vi "Intellirupter_coordinated.vi"() -> ()   [LabVIEW 2016]
uses:
  <vilib>/addons/Electrical Power/Protection/Definite Time Delay/subVIs/fpga_Time Delay Cfg.ctl
  <vilib>/FPGAPlugInAG/cRIO-9039 (Sync)/niLvFpga_Open_cRIO-9039 (Sync).vi
  <vilib>/rvi/interface/common/dynamic/niFpgaDynamicAddResources.vi
  <vilib>/Utility/error.llb/Error Cluster From Error Code.vi
  <vilib>/rvi/errors/niLvFpgaAdjustHostInterfaceError.vi
  <vilib>/FPGAPlugInAG/Dynamic/niLvFpga_Close_Dynamic.vi
  <vilib>/rvi/interface/nirviOpenFPGA/nirviOpenFPGA.xnode
  FPGA Bitfiles/IntelliRupter_calibrated.lvbitx
  <vilib>/rvi/interface/nirviReadWriteControl/nirviReadWriteControl.xnode
  <vilib>/rvi/interface/nirviCloseFPGA/nirviCloseFPGA.xnode
  <vilib>/rvi/interface/Simulation/niFpgaSimulationCallBeginRW.vi
  NiFpgaLv.dll
  <vilib>/addons/Electrical Power/Protection/NI_EP_Protection_FPGA.lvlib
panel:
  out "Block Relay8":bool
  out "Block Relay7":bool
  out "Block Relay5":bool
  out "Block Relay4":bool
  out "Block Relay2":bool
  out "Relay8\nBlocking signal":bool[](array[boolean])
  out "Relay7\nBlocking signal":bool[](array[boolean])
  out "Relay5\nBlocking signal":bool[](array[boolean])
  out "Relay4\nBlocking signal":bool[](array[boolean])
  out "Relay2\nBlocking signal":bool[](array[boolean])
  out "Trip Relay8":bool=TRUE
  out "Trip Relay7":bool
  out "Trip Relay6":bool=TRUE
  out "Trip Relay5":bool
  out "Trip Relay4":bool
  out "Trip Relay3":bool=TRUE
  out "Trip Relay2":bool
  out "Trip Relay1":bool
  out "MGCC_to_relay":bool[](array[boolean])=[TRUE, TRUE, FALSE, TRUE, TRUE, FALSE, TRUE, FALSE]
  out "Waveform Chart":dbl(graph)=-0.9071295261383057
  in  "Count(ticks)":u32=10000
  in  "RMS minimum\nvalues":T1={"VRMS values"=[0.5, 0.5, 0.5], "IRMS values"=[0.1, 0.1, 0.1]}
  out "error out":errorcluster
  out "Relay_toMGCC":bool[](array[boolean])=[TRUE, TRUE, FALSE, TRUE, TRUE, FALSE, TRUE, FALSE]
  in  "Manual trip Relay8":bool
  in  "Reclose Relay8?":bool
  out "R8 Data for\ncommunication":dbl[](array[numeric])=[0.0, 2.5009880757512857, 0.03119550342674121, 62.02715630655697, 302.3426407252326, -12.251248359680176, 0.16879604920390107, -0.031540152322164054, 0.0, 0.0]
  in  "Manual trip Relay7":bool
  in  "Reclose Relay7?":bool=TRUE
  out "R7 Data for\ncommunication":dbl[](array[numeric])=[0.0, 2.34510372262792, 2.478950931547994, 62.02269358678421, 62.00633268068818, -0.9071295261383057, 0.09051019032934479, -0.051861350624233596, 0.0, 0.0]
  in  "Manual trip Relay6":bool
  in  "Reclose Relay6?":bool
  out "R6 Data for\ncommunication":dbl[](array[numeric])=[0.0, 2.348051907862318, 0.01545718535019481, 62.01511039984677, 317.9551888289113, -12.64305591583252, 0.014835873481385646, -0.011305832700669725, 0.0, 0.0]
  in  "Manual trip Relay5":bool
  in  "Reclose Relay5?":bool=TRUE
  out "R5 Data for\ncommunication":dbl[](array[numeric])=[1.0, 2.346495418202577, 2.356958918684434, 62.01843298132032, 62.025906318306994, -0.8903157114982605, -0.5565142908906333, -0.4184036072959372, 0.0, 0.0]
  in  "Manual trip Relay4":bool
  in  "Reclose Relay4?":bool=TRUE
  out "R4 Data for\ncommunication":dbl[](array[numeric])=[1.0, 2.35949711967503, 2.3520019383369224, 62.03276424249066, 62.0133797943195, -0.28130459785461426, 0.5952503478367136, 0.39746847420084586, 0.0, 0.0]
  in  "Manual trip Relay3":bool
  in  "Reclose Relay3?":bool
  out "R3 Data for\ncommunication":dbl[](array[numeric])=[0.0, 2.3645958826384064, 0.01384802207001256, 62.02232220042387, 281.0580123337938, 37.610870361328125, 0.01240386848085533, 0.025416571188110054, 0.0, 0.0]
  in  "Manual trip Relay2":bool
  in  "Reclose Relay2?":bool=TRUE
  out "R2 Data for\ncommunication":dbl[](array[numeric])=[1.0, 2.35591902204862, 2.357236343046619, 62.02966341388489, 62.010588677473145, 0.21399852633476257, 1.122459889869548, 0.5804481897422749, 0.0, 0.0]
  out "R1 Data for\ncommunication":dbl[](array[numeric])=[1.0, 2.364986795195867, 2.3598010106583396, 62.02800601231562, 62.01433053877221, 0.17643588781356812, 1.6919416172136679, 0.8721834487461031, 0.0, 0.0]
  in  "Relay8":bool
  in  "Relay7":bool
  in  "Relay6":bool
  in  "Relay5":bool=TRUE
  in  "Relay4":bool=TRUE
  in  "Relay3":bool
  in  "Relay2":bool=TRUE
  in  "Reclose Relay1?":bool=TRUE
  out "half cycle (samples)":i32=96
  out "basic calc interval":u16=2074
  in  "stop":bool
  in  "Relay1":bool=TRUE
  in  "Manual trip Relay1":bool
  # "status\nmag_left\nmag_right\nfreq_left\nfreq_right\nang_diff\nact_power\nrea_power\n0\n0"
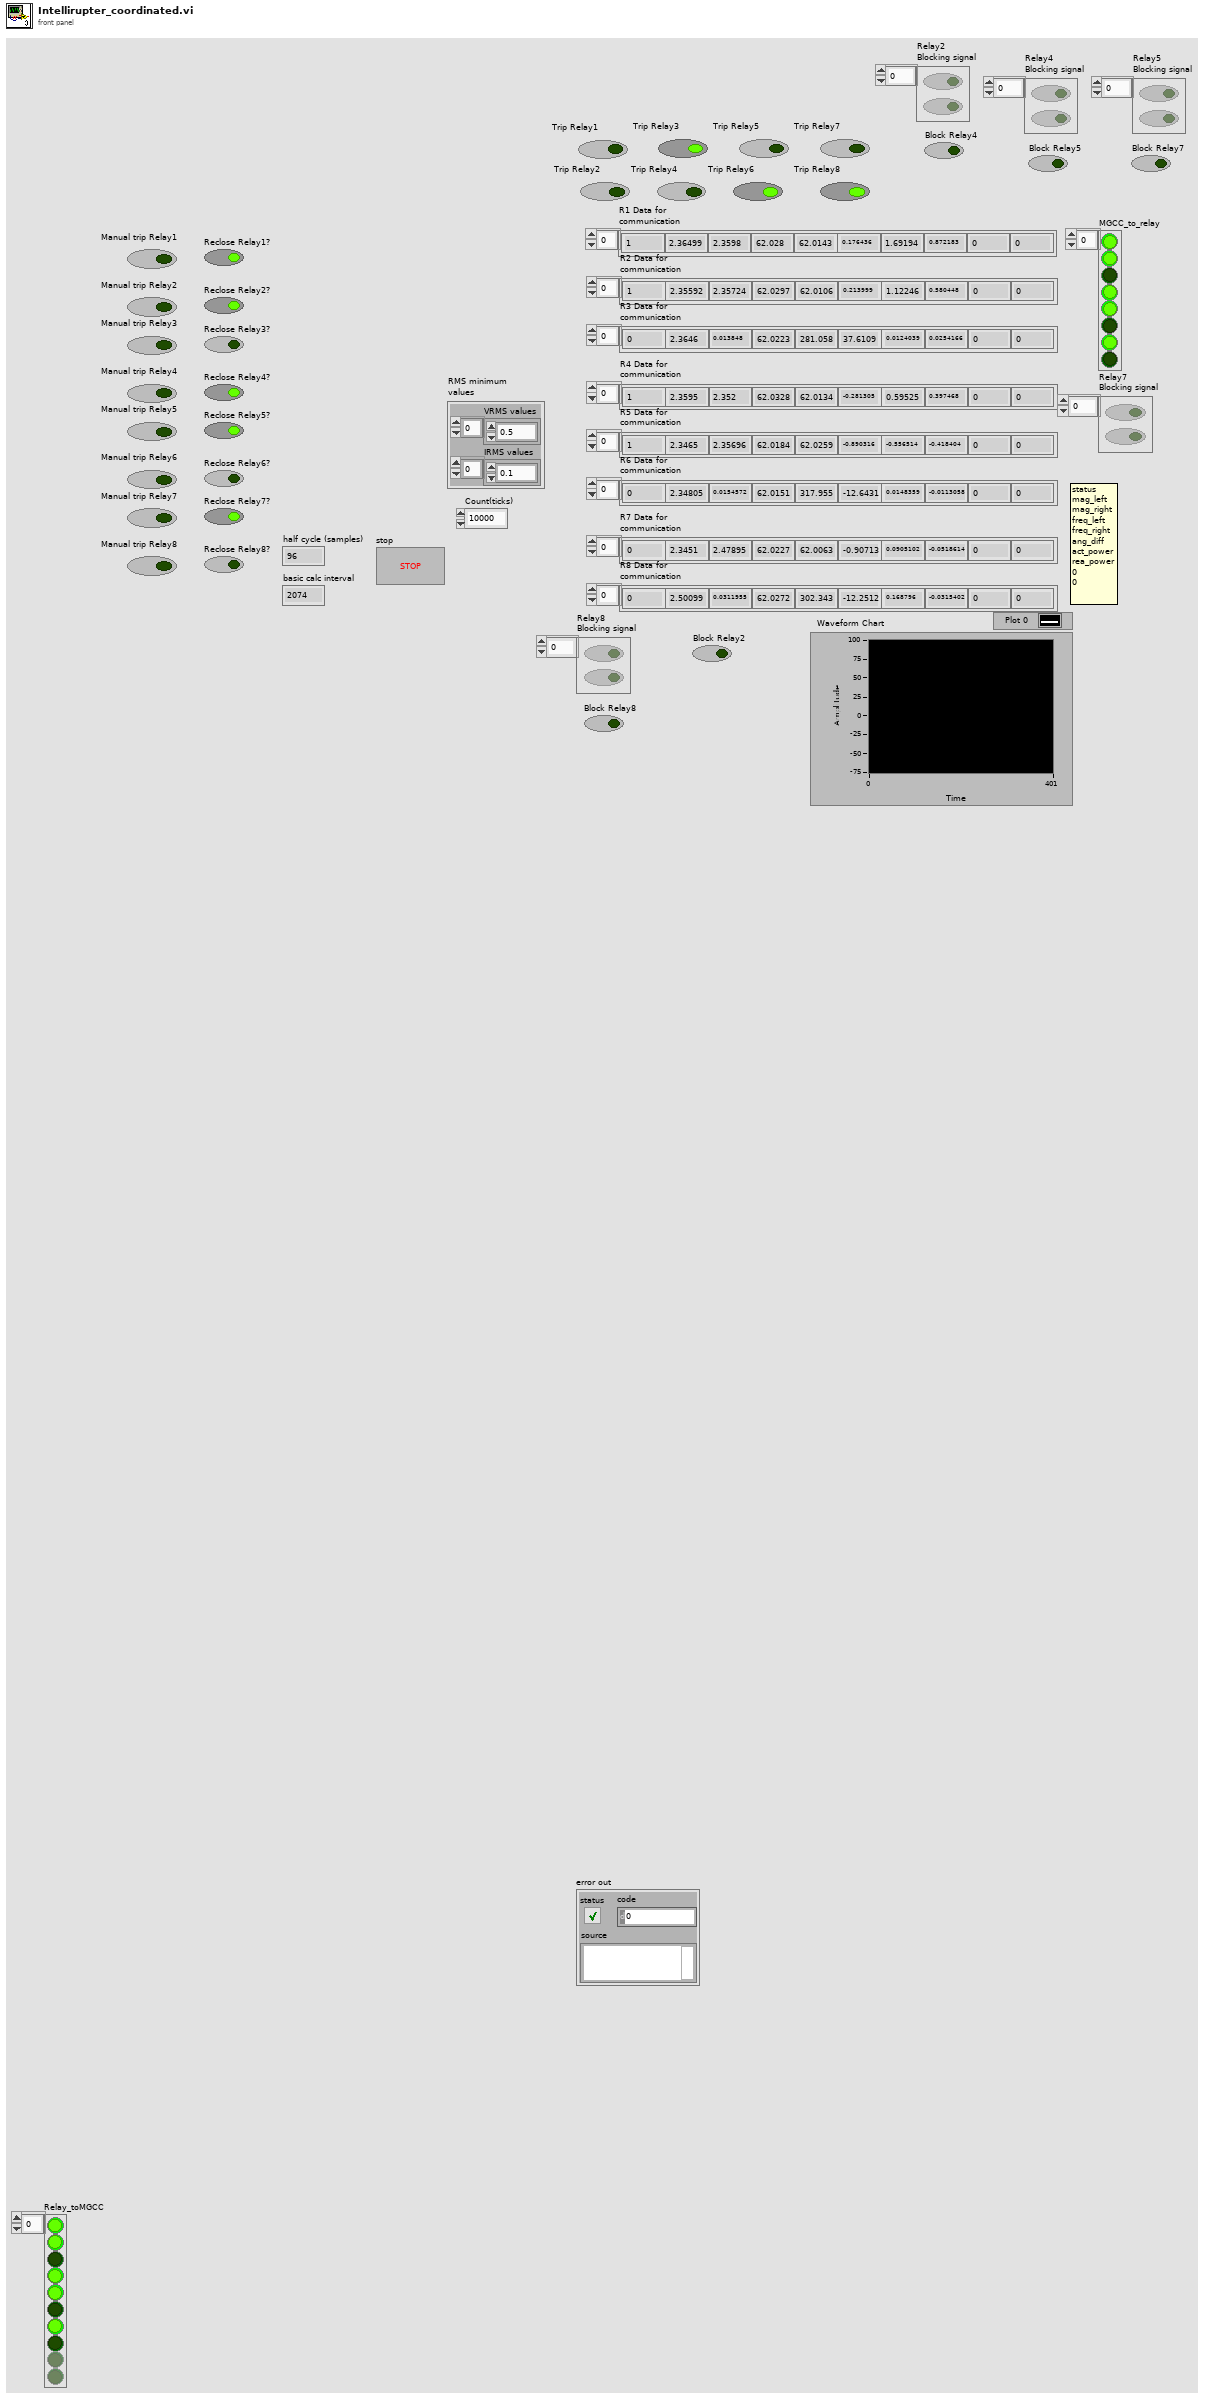
[diagram p1: front panel]
types:
  T1 = cluster{"VRMS values":dbl[], "IRMS values":dbl[]}
  T2 = cluster{fxp<+/-,53,11>[], fxp<+/-,53,11>[], fxp<+/-,53,11>[], fxp<+/-,53,11>[], fxp<+/-,53,11>[], fxp<+/-,53,11>[], fxp<+/-,53,11>[], fxp<+/-,53,11>[], fxp<+/-,53,11>[]}
  T3 = typedef "NI_EP_Protection_FPGA.lvlib/fpga_Time Delay Cfg.ctl" = cluster{"operate time [ms]":u32, "reset time [ms]":u32, "operate time compensation [ms]":u32}
  T4 = cluster{"UV Reset level":dbl, "Undervoltage \npick-up level":dbl, "OC Reset level":dbl, "Overcurrent\npick-up level":dbl, "time delay settings":T3}
  T5 = cluster{"Magnitude Minimum":dbl, "Magnitude difference level":dbl, "Frequency difference level":dbl, "Phase difference level":dbl}
  T6 = cluster{"RMS values":dbl[], "RMS values":dbl[], "RMS values":dbl[]}
  T7 = typedef "NI_EP_Protection_FPGA.lvlib/fpga_Timer Feedback Var.ctl" = cluster{"time elapsed":u32, "start time of trip counting":u32, "start time of reseting":u32}
  T8 = typedef "NI_EP_Protection_FPGA.lvlib/fpga_State.ctl" = enum16{"Idle", "Trip Counting", "Tripped", "Reset Counting"}
  T9 = cluster{bool, bool, "Boolean":bool, "timing values out":T7, "status out":T8, "trip signal out":bool}
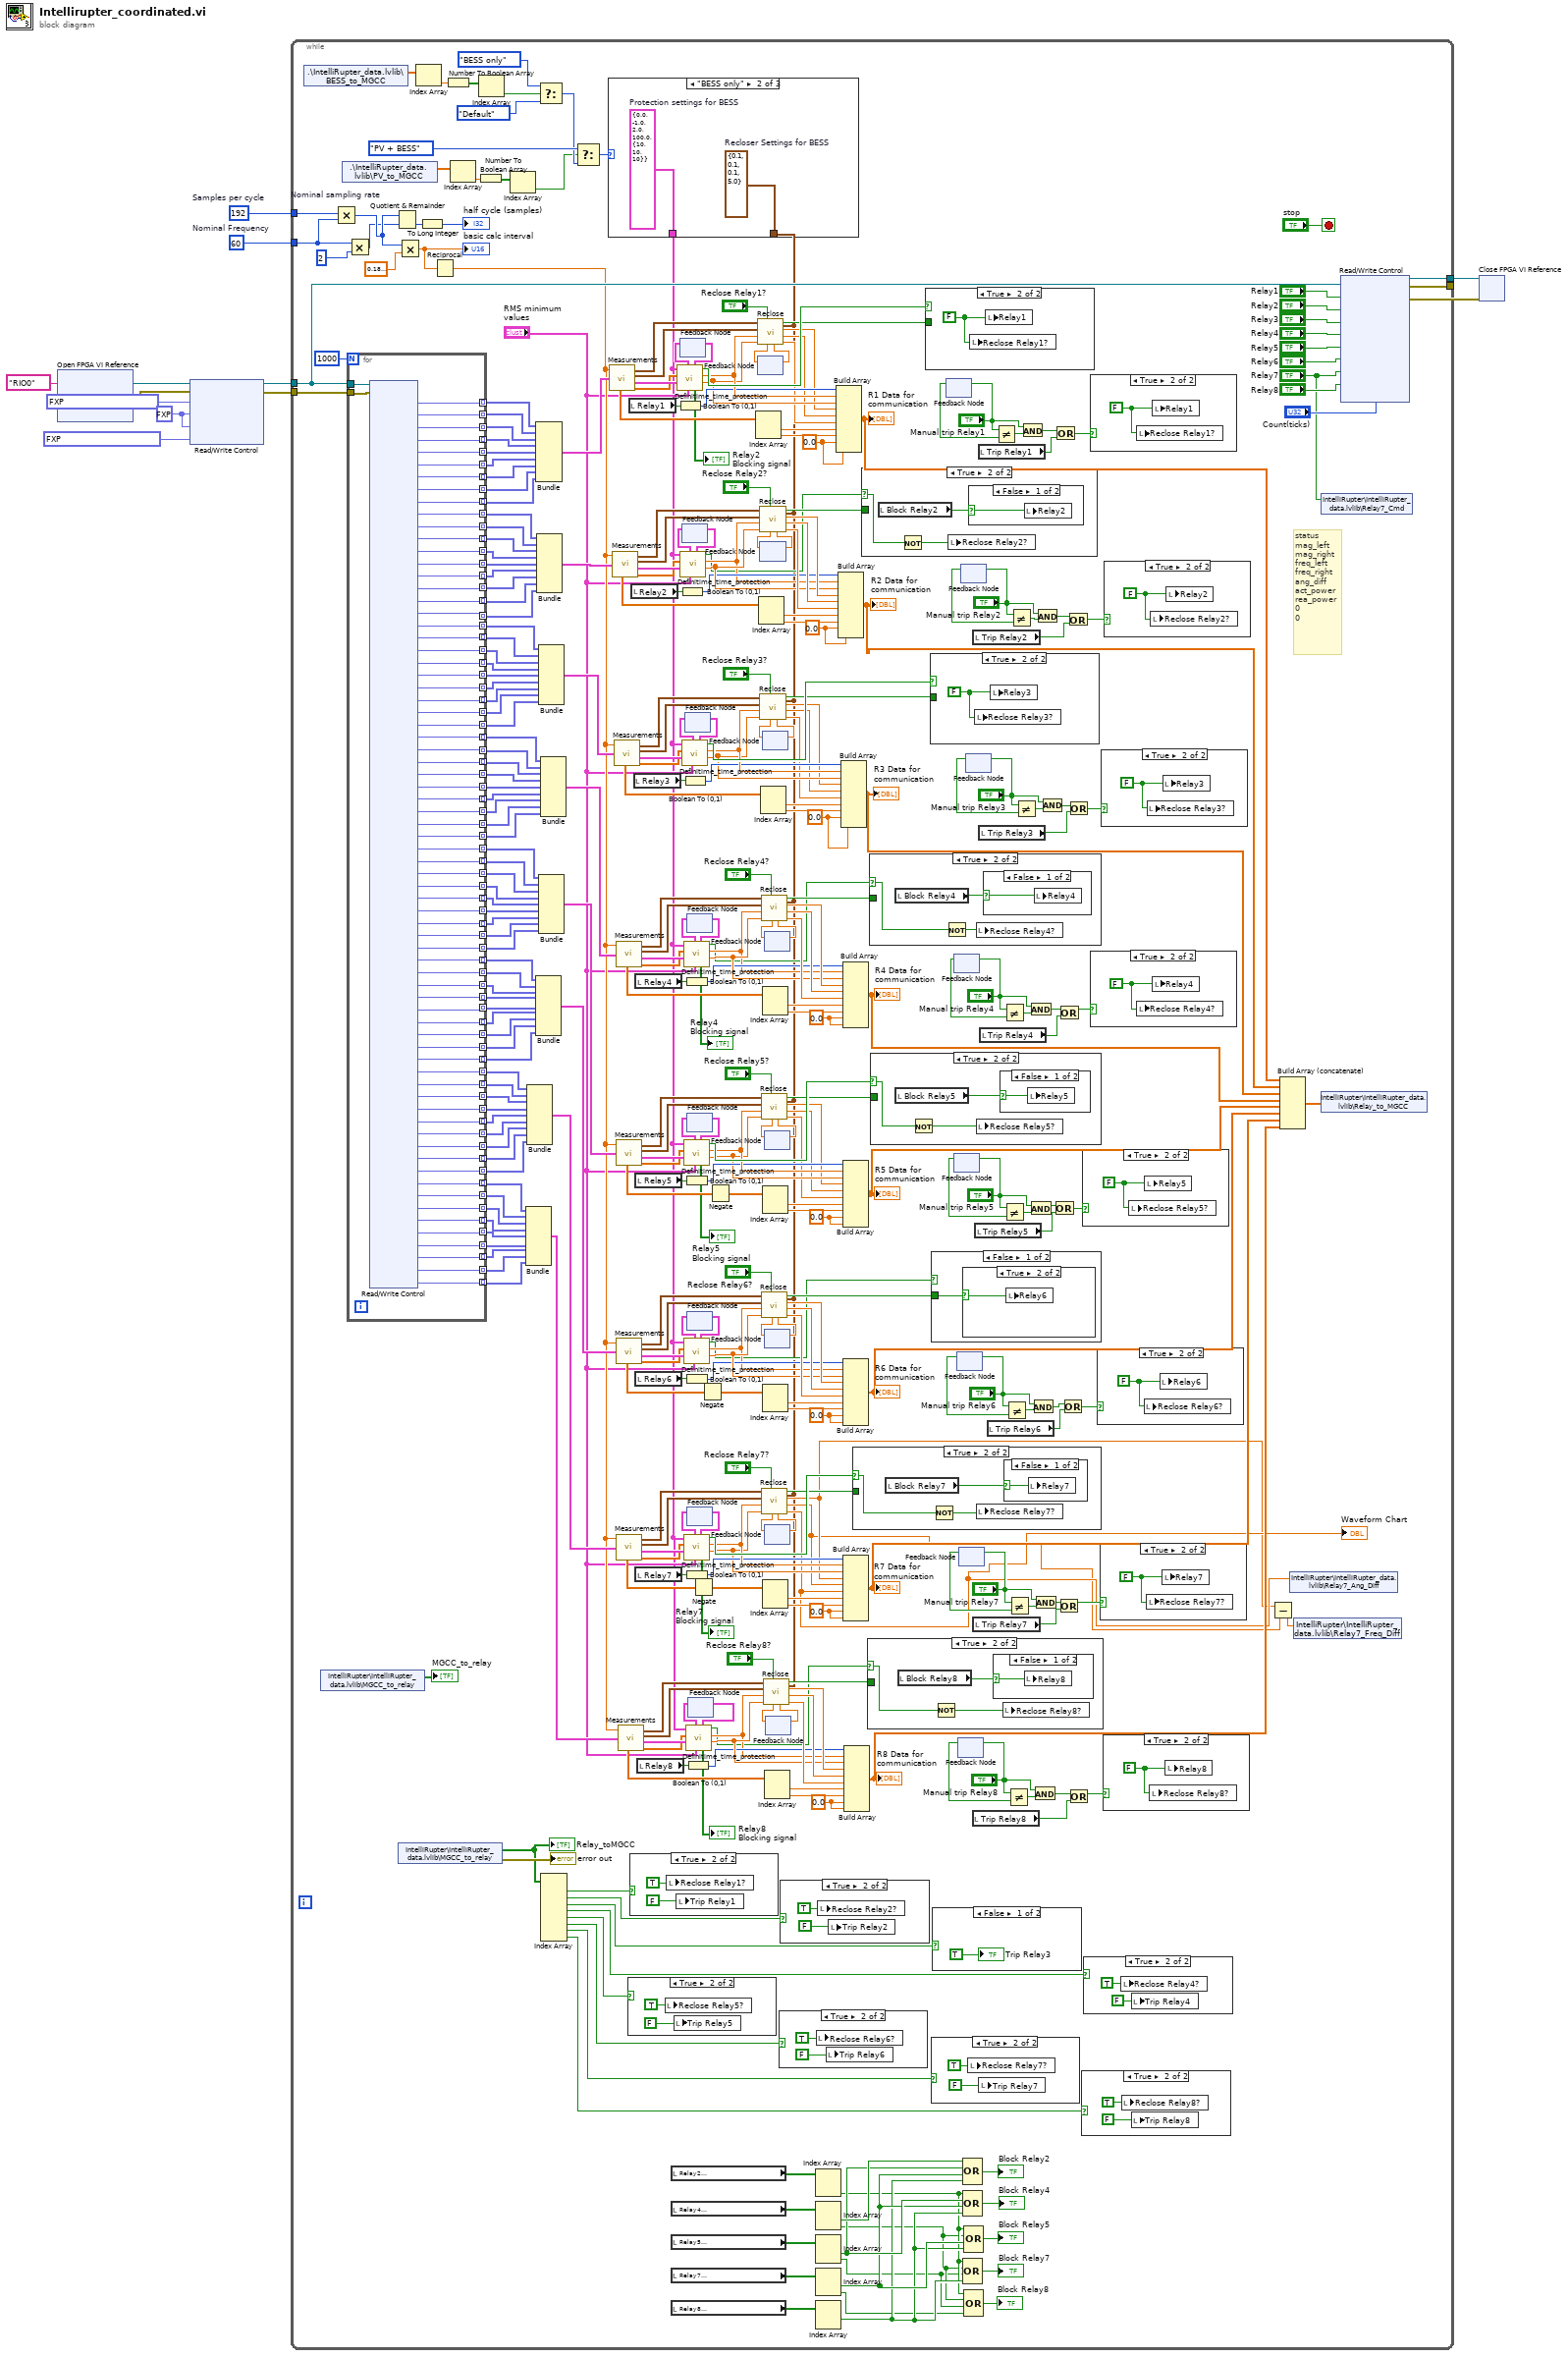
[diagram p0: block diagram]
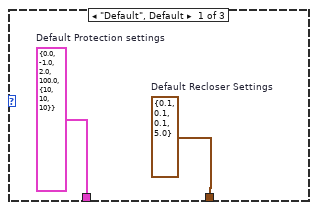
[diagram p2: hidden frame]
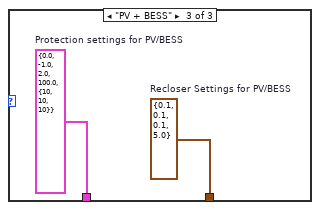
[diagram p3: hidden frame]
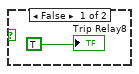
[diagram p4: hidden frame]
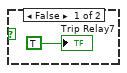
[diagram p5: hidden frame]
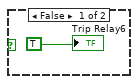
[diagram p6: hidden frame]
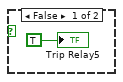
[diagram p7: hidden frame]
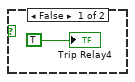
[diagram p8: hidden frame]
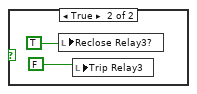
[diagram p9: hidden frame]
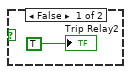
[diagram p10: hidden frame]
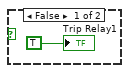
[diagram p11: hidden frame]
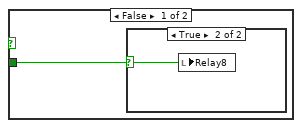
[diagram p12: hidden frame]
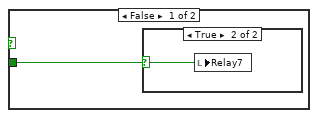
[diagram p16: hidden frame]
diagram:
  w2 = fxp<+/-,52,10> 0.0 ("I offset")
  w1 = 192  # Samples per cycle
  w10 = 60  # Nominal Frequency
  n1 = xnode "Open FPGA VI Reference"("resource name"=tag "RIO0") -> ("FPGA VI Reference Out"=w12:refnum<k20>, "error out"=w6:errorcluster)  [unwired: 1 in]
  n2 = xnode "Read/Write Control"("FPGA VI Reference In"=w12, "error in"=w6, "I scale factor"=fxp<+/-,26,5> 0.4499998092651367, "I offset"=w2, "V offset"=w2, "V scale factor"=fxp<+/-,26,5> 0.40000009536743164) -> ("FPGA VI Reference Out"=w7:refnum<k20>, "error out"=w5:errorcluster)
  n3 = while {
    tunnel: w7 -> [w389]
    tunnel: w10 -> [w397]
    tunnel: [w395] -> w9
    tunnel: [w394] -> w8
    tunnel: w5 -> [w388]
    tunnel: w1 -> [w96]
    stop <- "stop" stop-if-true
    w134 = 0.0 ("element")
    w145 = 0.0 ("element")
    w200 = 0.0 ("element")
    w211 = 0.0 ("element")
    w279 = 0.0 ("element")
    w289 = 0.0 ("element")
    w339 = 0.0 ("element")
    w355 = 0.0 ("element")
    # "status\nmag_left\nmag_right\nfreq_left\nfreq_right\nang_diff\nact_power\nrea_power\n0\n0"
    n4 = shared-variable ".\\IntelliRupter_data.lvlib\\BESS_to_MGCC"() -> (w37:dbl[])  [unwired: 1 in, 1 out]
    n5 = shared-variable "IntelliRupter\\IntelliRupter_data.lvlib\\MGCC_to_relay"() -> (→"MGCC_to_relay":bool[])  [unwired: 1 in, 1 out]
    n6 = Multiply "Nominal sampling rate"(x=w96, y=w397) -> (x*y=w403:i32)
    n7 = shared-variable ".\\IntelliRupter_data.lvlib\\PV_to_MGCC"() -> (w41:dbl[])  [unwired: 1 in, 1 out]
    n8 = Multiply(x=w397, y=2) -> (x*y=w399:i32)
    n9 = for {
      N: 1000 -> [_]
      tunnel: w389 -> [w551]
      tunnel: w388 -> [w550]
      tunnel: [w549] -> w386 mode=indexing
      tunnel: [w548] -> w385 mode=indexing
      tunnel: [w547] -> w384 mode=indexing
      tunnel: [w546] -> w383 mode=indexing
      tunnel: [w545] -> w382 mode=indexing
      tunnel: [w544] -> w381 mode=indexing
      tunnel: [w543] -> w380 mode=indexing
      tunnel: [w542] -> w379 mode=indexing
      tunnel: [w541] -> w378 mode=indexing
      tunnel: [w540] -> w348 mode=indexing
      tunnel: [w539] -> w347 mode=indexing
      tunnel: [w538] -> w346 mode=indexing
      tunnel: [w537] -> w345 mode=indexing
      tunnel: [w536] -> w344 mode=indexing
      tunnel: [w535] -> w343 mode=indexing
      tunnel: [w534] -> w342 mode=indexing
      tunnel: [w533] -> w341 mode=indexing
      tunnel: [w532] -> w340 mode=indexing
      tunnel: [w531] -> w288 mode=indexing
      tunnel: [w530] -> w287 mode=indexing
      tunnel: [w529] -> w286 mode=indexing
      tunnel: [w528] -> w285 mode=indexing
      tunnel: [w527] -> w284 mode=indexing
      tunnel: [w526] -> w283 mode=indexing
      tunnel: [w525] -> w282 mode=indexing
      tunnel: [w524] -> w281 mode=indexing
      tunnel: [w523] -> w280 mode=indexing
      tunnel: [w522] -> w253 mode=indexing
      tunnel: [w521] -> w252 mode=indexing
      tunnel: [w520] -> w251 mode=indexing
      tunnel: [w519] -> w250 mode=indexing
      tunnel: [w518] -> w249 mode=indexing
      tunnel: [w517] -> w248 mode=indexing
      tunnel: [w516] -> w247 mode=indexing
      tunnel: [w515] -> w246 mode=indexing
      tunnel: [w514] -> w245 mode=indexing
      tunnel: [w513] -> w244 mode=indexing
      tunnel: [w512] -> w243 mode=indexing
      tunnel: [w511] -> w242 mode=indexing
      tunnel: [w510] -> w241 mode=indexing
      tunnel: [w509] -> w240 mode=indexing
      tunnel: [w508] -> w239 mode=indexing
      tunnel: [w507] -> w238 mode=indexing
      tunnel: [w506] -> w237 mode=indexing
      tunnel: [w505] -> w236 mode=indexing
      tunnel: [w504] -> w209 mode=indexing
      tunnel: [w503] -> w208 mode=indexing
      tunnel: [w502] -> w207 mode=indexing
      tunnel: [w501] -> w206 mode=indexing
      tunnel: [w500] -> w205 mode=indexing
      tunnel: [w499] -> w204 mode=indexing
      tunnel: [w498] -> w203 mode=indexing
      tunnel: [w497] -> w202 mode=indexing
      tunnel: [w496] -> w201 mode=indexing
      tunnel: [w495] -> w174 mode=indexing
      tunnel: [w494] -> w173 mode=indexing
      tunnel: [w493] -> w172 mode=indexing
      tunnel: [w492] -> w171 mode=indexing
      tunnel: [w491] -> w170 mode=indexing
      tunnel: [w490] -> w169 mode=indexing
      tunnel: [w489] -> w168 mode=indexing
      tunnel: [w488] -> w167 mode=indexing
      tunnel: [w487] -> w166 mode=indexing
      tunnel: [w486] -> w143 mode=indexing
      tunnel: [w485] -> w142 mode=indexing
      tunnel: [w484] -> w141 mode=indexing
      tunnel: [w483] -> w140 mode=indexing
      tunnel: [w482] -> w139 mode=indexing
      tunnel: [w481] -> w138 mode=indexing
      tunnel: [w480] -> w137 mode=indexing
      tunnel: [w479] -> w136 mode=indexing
      tunnel: [w478] -> w135 mode=indexing
      n10 = xnode "Read/Write Control"("FPGA VI Reference In"=w551, "error in"=w550) -> ("V1L AB"=w549:fxp<+/-,53,11>, "V1L BC"=w548:fxp<+/-,53,11>, "V1L CA"=w547:fxp<+/-,53,11>, "V1R AB"=w546:fxp<+/-,53,11>, "V1R BC"=w545:fxp<+/-,53,11>, "V1R CA"=w544:fxp<+/-,53,11>, "I1 A"=w543:fxp<+/-,53,11>, "I1 B"=w542:fxp<+/-,53,11>, "I1 C"=w541:fxp<+/-,53,11>, "V2L AB"=w540:fxp<+/-,53,11>, "V2L BC"=w539:fxp<+/-,53,11>, "V2L CA"=w538:fxp<+/-,53,11>, "V2R AB"=w537:fxp<+/-,53,11>, "V2R BC"=w536:fxp<+/-,53,11>, "V2R CA"=w535:fxp<+/-,53,11>, "I2 A"=w534:fxp<+/-,53,11>, "I2 B"=w533:fxp<+/-,53,11>, "I2 C"=w532:fxp<+/-,53,11>, "V3L AB"=w531:fxp<+/-,53,11>, "V3L BC"=w530:fxp<+/-,53,11>, "V3L CA"=w529:fxp<+/-,53,11>, "V3R AB"=w528:fxp<+/-,53,11>, "V3R BC"=w527:fxp<+/-,53,11>, "V3R CA"=w526:fxp<+/-,53,11>, "I3 A"=w525:fxp<+/-,53,11>, "I3 B"=w524:fxp<+/-,53,11>, "I3 C"=w523:fxp<+/-,53,11>, "V4L AB"=w522:fxp<+/-,53,11>, "V4L BC"=w521:fxp<+/-,53,11>, "V4L CA"=w520:fxp<+/-,53,11>, "V4R AB"=w519:fxp<+/-,53,11>, "V4R BC"=w518:fxp<+/-,53,11>, "V4R CA"=w517:fxp<+/-,53,11>, "I4 A"=w516:fxp<+/-,53,11>, "I4 B"=w515:fxp<+/-,53,11>, "I4 C"=w514:fxp<+/-,53,11>, "V5L AB"=w513:fxp<+/-,53,11>, "V5L BC"=w512:fxp<+/-,53,11>, "V5L CA"=w511:fxp<+/-,53,11>, "V5R AB"=w510:fxp<+/-,53,11>, "V5R BC"=w509:fxp<+/-,53,11>, "V5R CA"=w508:fxp<+/-,53,11>, "I5 A"=w507:fxp<+/-,53,11>, "I5 B"=w506:fxp<+/-,53,11>, "I5 C"=w505:fxp<+/-,53,11>, "V6L AB"=w504:fxp<+/-,53,11>, "V6L BC"=w503:fxp<+/-,53,11>, "V6L CA"=w502:fxp<+/-,53,11>, "V6R AB"=w501:fxp<+/-,53,11>, "V6R BC"=w500:fxp<+/-,53,11>, "V6R CA"=w499:fxp<+/-,53,11>, "I6 A"=w498:fxp<+/-,53,11>, "I6 B"=w497:fxp<+/-,53,11>, "I6 C"=w496:fxp<+/-,53,11>, "V7L AB"=w495:fxp<+/-,53,11>, "V7L BC"=w494:fxp<+/-,53,11>, "V7L CA"=w493:fxp<+/-,53,11>, "V7R AB"=w492:fxp<+/-,53,11>, "V7R BC"=w491:fxp<+/-,53,11>, "V7R CA"=w490:fxp<+/-,53,11>, "I7 A"=w489:fxp<+/-,53,11>, "I7 B"=w488:fxp<+/-,53,11>, "I7 C"=w487:fxp<+/-,53,11>, "V8L AB"=w486:fxp<+/-,53,11>, "V8L BC"=w485:fxp<+/-,53,11>, "V8L CA"=w484:fxp<+/-,53,11>, "V8R AB"=w483:fxp<+/-,53,11>, "V8R BC"=w482:fxp<+/-,53,11>, "V8R CA"=w481:fxp<+/-,53,11>, "I8 A"=w480:fxp<+/-,53,11>, "I8 B"=w479:fxp<+/-,53,11>, "I8 C"=w478:fxp<+/-,53,11>)  [unwired: 2 out]
    }
    n11 = Quotient & Remainder(x=w403, y=w399) -> (floor(x/y)=w401:i32)  [unwired: 1 out]
    n12 = Multiply(x=w403, y=sgl 0.18) -> (x*y=w404:sgl)
    "basic calc interval" <- w404
    n13 = shared-variable "IntelliRupter\\IntelliRupter_data.lvlib\\MGCC_to_relay"() -> (w91:bool[], error out=→"error out":errorcluster)  [unwired: 1 in]
    "Relay_toMGCC" <- w91
    n14 = Index Array(array=w37) -> (element=w36:dbl)  [unwired: 1 in]
    n15 = To Long Integer(number=w401) -> (32bit integer=→"half cycle (samples)":i32)
    n16 = Reciprocal(x=w404) -> (1/x=w109:sgl)
    n17 = Number To Boolean Array(number=w36) -> (Boolean array=w45:bool[])
    n18 = Index Array(array=w41) -> (element=w40:dbl)  [unwired: 1 in]
    n19 = Number To Boolean Array(number=w40) -> (Boolean array=w39:bool[])
    n20 = Index Array(array=w45) -> (element=w44:bool)  [unwired: 1 in]
    n21 = Index Array(array=w39) -> (element=w38:bool)  [unwired: 1 in]
    n22 = Bundle(w143, w142, w141, w140, w139, w138, w137, w136, w135) -> (w108:T2)  [unwired: 1 in]
    n23 = Bundle(w174, w173, w172, w171, w170, w169, w168, w167, w166) -> (w144:T2)  [unwired: 1 in]
    n24 = Bundle(w209, w208, w207, w206, w205, w204, w203, w202, w201) -> (w176:T2)  [unwired: 1 in]
    n25 = Bundle(w386, w385, w384, w383, w382, w381, w380, w379, w378) -> (w377:T2)  [unwired: 1 in]
    n26 = Bundle(w348, w347, w346, w345, w344, w343, w342, w341, w340) -> (w314:T2)  [unwired: 1 in]
    n27 = Select(t=enum16{"Default", "BESS only", "PV + BESS"}."BESS only", s=w44, f=enum16{"Default", "BESS only", "PV + BESS"}."Default") -> (s? t:f=w46:enum16{"Default", "BESS only", "PV + BESS"})
    n28 = Bundle(w288, w287, w286, w285, w284, w283, w282, w281, w280) -> (w313:T2)  [unwired: 1 in]
    n29 = Bundle(w244, w243, w242, w241, w240, w239, w238, w237, w236) -> (w210:T2)  [unwired: 1 in]
    n30 = Bundle(w253, w252, w251, w250, w249, w248, w247, w246, w245) -> (w254:T2)  [unwired: 1 in]
    n31 = Index Array(array=w91) -> (element #1=w90:bool, element #2=w89:bool, element #3=w88:bool, element #4=w87:bool, element #5=w86:bool, element #6=w85:bool, element #7=w84:bool, element #8=w83:bool)  [unwired: 8 in]
    n32 = Select(t=enum16{"Default", "BESS only", "PV + BESS"}."PV + BESS", s=w38, f=w46) -> (s? t:f=w48:enum16{"Default", "BESS only", "PV + BESS"})
    n33 = case shown="\"BESS only\"" w48 {
      tunnel: [w405 w408 w409] -> w50
      tunnel: [w406 w407 w410] -> w49
      frame "Default", Default {
        w406 = T4 {"UV Reset level"=0.0, "Undervoltage \npick-up level"=-1.0, "OC Reset level"=2.0, "Overcurrent\npick-up level"=100.0, "time delay settings"={"operate time [ms]"=10, "reset time [ms]"=10, "operate time compensation [ms]"=10}}  # Default Protection settings
        w405 = T5 {"Magnitude Minimum"=0.1, "Magnitude difference level"=0.1, "Frequency difference level"=0.1, "Phase difference level"=5.0}  # Default Recloser Settings
      }
      frame "BESS only" {
        w407 = T4 {"UV Reset level"=0.0, "Undervoltage \npick-up level"=-1.0, "OC Reset level"=2.0, "Overcurrent\npick-up level"=100.0, "time delay settings"={"operate time [ms]"=10, "reset time [ms]"=10, "operate time compensation [ms]"=10}}  # Protection settings for BESS
        w408 = T5 {"Magnitude Minimum"=0.1, "Magnitude difference level"=0.1, "Frequency difference level"=0.1, "Phase difference level"=5.0}  # Recloser Settings for BESS
      }
      frame "PV + BESS" {
        w410 = T4 {"UV Reset level"=0.0, "Undervoltage \npick-up level"=-1.0, "OC Reset level"=2.0, "Overcurrent\npick-up level"=100.0, "time delay settings"={"operate time [ms]"=10, "reset time [ms]"=10, "operate time compensation [ms]"=10}}  # Protection settings for PV/BESS
        w409 = T5 {"Magnitude Minimum"=0.1, "Magnitude difference level"=0.1, "Frequency difference level"=0.1, "Phase difference level"=5.0}  # Recloser Settings for PV/BESS
      }
    }
    n34 = call "Measurements.vi"("dt"=w109, "Input cluster"=w377) -> ("Total power values"=w358:dbl[], "VL array"=w375:waveform(sgl)[], "VR array"=w374:waveform(sgl)[], "RMS values"=w376:T6, "Active Power"=w66:dbl[])  [unwired: 2 in]
    n35 = call "Measurements.vi"("dt"=w109, "Input cluster"=w314) -> ("Total power values"=w336:dbl[], "VL array"=w320:waveform(sgl)[], "VR array"=w321:waveform(sgl)[], "RMS values"=w319:T6, "Active Power"=w65:dbl[])  [unwired: 2 in]
    n36 = call "Measurements.vi"("dt"=w109, "Input cluster"=w313) -> ("Total power values"=w291:dbl[], "VL array"=w307:waveform(sgl)[], "VR array"=w306:waveform(sgl)[], "RMS values"=w308:T6, "Active Power"=w64:dbl[])  [unwired: 2 in]
    n37 = call "Measurements.vi"("dt"=w109, "Input cluster"=w254) -> ("Total power values"=w276:dbl[], "VL array"=w260:waveform(sgl)[], "VR array"=w261:waveform(sgl)[], "RMS values"=w259:T6, "Active Power"=w63:dbl[])  [unwired: 2 in]
    n38 = call "Measurements.vi"("dt"=w109, "Input cluster"=w210) -> ("Total power values"=w214:dbl[], "VL array"=w230:waveform(sgl)[], "VR array"=w229:waveform(sgl)[], "RMS values"=w231:T6, "Active Power"=w62:dbl[])  [unwired: 2 in]
    n39 = call "Measurements.vi"("dt"=w109, "Input cluster"=w176) -> ("Total power values"=w175:dbl[], "VL array"=w182:waveform(sgl)[], "VR array"=w183:waveform(sgl)[], "RMS values"=w181:T6, "Active Power"=w61:dbl[])  [unwired: 2 in]
    n40 = call "Measurements.vi"("dt"=w109, "Input cluster"=w144) -> ("Total power values"=w165:dbl[], "VL array"=w159:waveform(sgl)[], "VR array"=w158:waveform(sgl)[], "RMS values"=w160:T6, "Active Power"=w60:dbl[])  [unwired: 2 in]
    n41 = call "Measurements.vi"("dt"=w109, "Input cluster"=w108) -> ("Total power values"=w110:dbl[], "VL array"=w116:waveform(sgl)[], "VR array"=w117:waveform(sgl)[], "RMS values"=w115:T6, "Active Power"=w59:dbl[])  [unwired: 2 in]
    n42 = case shown="True" w86 {
      frame False {
        "Trip Relay5" <- TRUE ("Manual trip Relay1")
      }
      frame True {
        n43 = local write "Reclose Relay5?"(TRUE ("Reclose Relay1?")) -> ()
        n44 = local write "Trip Relay5"(FALSE ("Reclose Relay1?")) -> ()
      }
    }
    n45 = local read "Relay1"() -> (w365:bool)
    n46 = case shown="True" w90 {
      frame False {
        "Trip Relay1" <- TRUE ("Manual trip Relay1")
      }
      frame True {
        n47 = local write "Reclose Relay1?"(TRUE ("Reclose Relay1?")) -> ()
        n48 = local write "Trip Relay1"(FALSE ("Reclose Relay1?")) -> ()
      }
    }
    n49 = local read "Relay2"() -> (w329:bool)
    n50 = local read "Relay3"() -> (w298:bool)
    n51 = local read "Relay4"() -> (w269:bool)
    n52 = local read "Relay5"() -> (w221:bool)
    n53 = local read "Relay6"() -> (w191:bool)
    n54 = local read "Relay7"() -> (w150:bool)
    n55 = local read "Relay8"() -> (w125:bool)
    n56 = local read "Relay2\nBlocking signal"() -> (w30:bool[])
    n57 = local read "Relay4\nBlocking signal"() -> (w29:bool[])
    n58 = local read "Relay5\nBlocking signal"() -> (w28:bool[])
    n59 = local read "Relay7\nBlocking signal"() -> (w27:bool[])
    n60 = local read "Relay8\nBlocking signal"() -> (w26:bool[])
    n61 = Boolean To (0,1)(Boolean=w365) -> (0, 1=w363:i16)
    n62 = feedback #1() -> (w372:T9)  [unwired: 1 in]
    n63 = call "Definitime_time_protection.vi"("RMS minimum\nvalues"="RMS minimum\nvalues", "input cluster"=w372, "RMS values"=w376, "Active Power"=w66, "Protection settings"=w49) -> ("VR RMS"=w362:dbl, "VL RMS"=w364:dbl, "trip signal"=w368:bool, "Blocking signal"=→"Relay2\nBlocking signal":bool[], "output cluster"=w373:T9)  [unwired: 1 in, 1 out]
    n64 = feedback-in #1(w373) -> ()
    n65 = Boolean To (0,1)(Boolean=w329) -> (0, 1=w331:i16)
    n66 = feedback #2() -> (w323:T9)  [unwired: 1 in]
    n67 = call "Definitime_time_protection.vi"("RMS minimum\nvalues"="RMS minimum\nvalues", "input cluster"=w323, "RMS values"=w319, "Active Power"=w65, "Protection settings"=w49) -> ("VR RMS"=w332:dbl, "VL RMS"=w330:dbl, "trip signal"=w327:bool, "output cluster"=w322:T9)  [unwired: 1 in, 2 out]
    n68 = feedback-in #2(w322) -> ()
    n69 = Boolean To (0,1)(Boolean=w298) -> (0, 1=w296:i16)
    n70 = Boolean To (0,1)(Boolean=w269) -> (0, 1=w271:i16)
    n71 = Boolean To (0,1)(Boolean=w221) -> (0, 1=w219:i16)
    n72 = Boolean To (0,1)(Boolean=w191) -> (0, 1=w193:i16)
    n73 = Boolean To (0,1)(Boolean=w150) -> (0, 1=w148:i16)
    n74 = feedback #3() -> (w304:T9)  [unwired: 1 in]
    n75 = call "Definitime_time_protection.vi"("RMS minimum\nvalues"="RMS minimum\nvalues", "input cluster"=w304, "RMS values"=w308, "Active Power"=w64, "Protection settings"=w49) -> ("VR RMS"=w295:dbl, "VL RMS"=w297:dbl, "trip signal"=w300:bool, "output cluster"=w305:T9)  [unwired: 1 in, 2 out]
    n76 = feedback-in #3(w305) -> ()
    n77 = Boolean To (0,1)(Boolean=w125) -> (0, 1=w127:i16)
    n78 = feedback #4() -> (w263:T9)  [unwired: 1 in]
    n79 = call "Definitime_time_protection.vi"("RMS minimum\nvalues"="RMS minimum\nvalues", "input cluster"=w263, "RMS values"=w259, "Active Power"=w63, "Protection settings"=w49) -> ("VR RMS"=w272:dbl, "VL RMS"=w270:dbl, "trip signal"=w267:bool, "Blocking signal"=→"Relay4\nBlocking signal":bool[], "output cluster"=w262:T9)  [unwired: 1 in, 1 out]
    n80 = feedback-in #4(w262) -> ()
    n81 = feedback #5() -> (w227:T9)  [unwired: 1 in]
    n82 = call "Definitime_time_protection.vi"("RMS minimum\nvalues"="RMS minimum\nvalues", "input cluster"=w227, "RMS values"=w231, "Active Power"=w62, "Protection settings"=w49) -> ("VR RMS"=w218:dbl, "VL RMS"=w220:dbl, "trip signal"=w223:bool, "Blocking signal"=→"Relay5\nBlocking signal":bool[], "output cluster"=w228:T9)  [unwired: 1 in, 1 out]
    n83 = feedback-in #5(w228) -> ()
    n84 = feedback #6() -> (w185:T9)  [unwired: 1 in]
    n85 = call "Definitime_time_protection.vi"("RMS minimum\nvalues"="RMS minimum\nvalues", "input cluster"=w185, "RMS values"=w181, "Active Power"=w61, "Protection settings"=w49) -> ("VR RMS"=w194:dbl, "VL RMS"=w192:dbl, "trip signal"=w189:bool, "output cluster"=w184:T9)  [unwired: 1 in, 2 out]
    n86 = feedback-in #6(w184) -> ()
    n87 = feedback #7() -> (w156:T9)  [unwired: 1 in]
    n88 = call "Definitime_time_protection.vi"("RMS minimum\nvalues"="RMS minimum\nvalues", "input cluster"=w156, "RMS values"=w160, "Active Power"=w60, "Protection settings"=w49) -> ("VR RMS"=w147:dbl, "VL RMS"=w149:dbl, "trip signal"=w152:bool, "Blocking signal"=→"Relay7\nBlocking signal":bool[], "output cluster"=w157:T9)  [unwired: 1 in, 1 out]
    n89 = feedback-in #7(w157) -> ()
    n90 = feedback #8() -> (w119:T9)  [unwired: 1 in]
    n91 = call "Definitime_time_protection.vi"("RMS minimum\nvalues"="RMS minimum\nvalues", "input cluster"=w119, "RMS values"=w115, "Active Power"=w59, "Protection settings"=w49) -> ("VR RMS"=w128:dbl, "VL RMS"=w126:dbl, "trip signal"=w123:bool, "Blocking signal"=→"Relay8\nBlocking signal":bool[], "output cluster"=w118:T9)  [unwired: 1 in, 1 out]
    n92 = feedback-in #8(w118) -> ()
    n93 = Negate(x=w165) -> (-x=w53:dbl[])
    n94 = Negate(x=w175) -> (-x=w52:dbl[])
    n95 = Negate(x=w214) -> (-x=w51:dbl[])
    n96 = Index Array(array=w358) -> (element #1=w357:dbl, element #2=w356:dbl)  [unwired: 2 in]
    n97 = feedback #9() -> (w370:dbl)  [unwired: 1 in]
    n98 = call "Reclose.vi"("Recloser Settings"=w50, "Counter In"=w370, "Reclose?"="Reclose Relay1?", "VR RMS avg"=w362, "VL RMS avg"=w364, "VR array"=w374, "VL array"=w375) -> ("Phase difference"=w359:dbl, "VR Frequency"=w360:dbl, "VL Frequency"=w361:dbl, "Recloser action"=w367:bool, "Counter Out"=w371:dbl)
    n99 = feedback-in #9(w371) -> ()
    n100 = Index Array(array=w336) -> (element #1=w337:dbl, element #2=w338:dbl)  [unwired: 2 in]
    n101 = feedback #10() -> (w325:dbl)  [unwired: 1 in]
    n102 = call "Reclose.vi"("Recloser Settings"=w50, "Counter In"=w325, "Reclose?"="Reclose Relay2?", "VR RMS avg"=w332, "VL RMS avg"=w330, "VR array"=w321, "VL array"=w320) -> ("Phase difference"=w335:dbl, "VR Frequency"=w334:dbl, "VL Frequency"=w333:dbl, "Recloser action"=w328:bool, "Counter Out"=w324:dbl)
    n103 = feedback-in #10(w324) -> ()
    n104 = Index Array(array=w291) -> (element #1=w95:dbl, element #2=w290:dbl)  [unwired: 2 in]
    n105 = feedback #11() -> (w302:dbl)  [unwired: 1 in]
    n106 = call "Reclose.vi"("Recloser Settings"=w50, "Counter In"=w302, "Reclose?"="Reclose Relay3?", "VR RMS avg"=w295, "VL RMS avg"=w297, "VR array"=w306, "VL array"=w307) -> ("Phase difference"=w292:dbl, "VR Frequency"=w293:dbl, "VL Frequency"=w294:dbl, "Recloser action"=w299:bool, "Counter Out"=w303:dbl)
    n107 = feedback-in #11(w303) -> ()
    n108 = Index Array(array=w276) -> (element #1=w277:dbl, element #2=w278:dbl)  [unwired: 2 in]
    n109 = Index Array(array=w51) -> (element #1=w213:dbl, element #2=w212:dbl)  [unwired: 2 in]
    n110 = Index Array(array=w52) -> (element #1=w198:dbl, element #2=w199:dbl)  [unwired: 2 in]
    n111 = Index Array(array=w53) -> (element #1=w94:dbl, element #2=w146:dbl)  [unwired: 2 in]
    n112 = feedback #12() -> (w265:dbl)  [unwired: 1 in]
    n113 = call "Reclose.vi"("Recloser Settings"=w50, "Counter In"=w265, "Reclose?"="Reclose Relay4?", "VR RMS avg"=w272, "VL RMS avg"=w270, "VR array"=w261, "VL array"=w260) -> ("Phase difference"=w275:dbl, "VR Frequency"=w274:dbl, "VL Frequency"=w273:dbl, "Recloser action"=w268:bool, "Counter Out"=w264:dbl)
    n114 = feedback-in #12(w264) -> ()
    n115 = feedback #13() -> (w225:dbl)  [unwired: 1 in]
    n116 = call "Reclose.vi"("Recloser Settings"=w50, "Counter In"=w225, "Reclose?"="Reclose Relay5?", "VR RMS avg"=w218, "VL RMS avg"=w220, "VR array"=w229, "VL array"=w230) -> ("Phase difference"=w215:dbl, "VR Frequency"=w216:dbl, "VL Frequency"=w217:dbl, "Recloser action"=w222:bool, "Counter Out"=w226:dbl)
    n117 = feedback-in #13(w226) -> ()
    n118 = feedback #14() -> (w187:dbl)  [unwired: 1 in]
    n119 = call "Reclose.vi"("Recloser Settings"=w50, "Counter In"=w187, "Reclose?"="Reclose Relay6?", "VR RMS avg"=w194, "VL RMS avg"=w192, "VR array"=w183, "VL array"=w182) -> ("Phase difference"=w197:dbl, "VR Frequency"=w196:dbl, "VL Frequency"=w195:dbl, "Recloser action"=w190:bool, "Counter Out"=w186:dbl)
    n120 = feedback-in #14(w186) -> ()
    n121 = feedback #15() -> (w154:dbl)  [unwired: 1 in]
    n122 = call "Reclose.vi"("Recloser Settings"=w50, "Counter In"=w154, "Reclose?"="Reclose Relay7?", "VR RMS avg"=w147, "VL RMS avg"=w149, "VR array"=w158, "VL array"=w159) -> ("Phase difference"=w58:dbl, "VR Frequency"=w56:dbl, "VL Frequency"=w57:dbl, "Recloser action"=w151:bool, "Counter Out"=w155:dbl)
    "Waveform Chart" <- w58
    n123 = feedback-in #15(w155) -> ()
    n124 = Index Array(array=w110) -> (element #1=w132:dbl, element #2=w133:dbl)  [unwired: 2 in]
    n125 = feedback #16() -> (w121:dbl)  [unwired: 1 in]
    n126 = call "Reclose.vi"("Recloser Settings"=w50, "Counter In"=w121, "Reclose?"="Reclose Relay8?", "VR RMS avg"=w128, "VL RMS avg"=w126, "VR array"=w117, "VL array"=w116) -> ("Phase difference"=w131:dbl, "VR Frequency"=w130:dbl, "VL Frequency"=w129:dbl, "Recloser action"=w124:bool, "Counter Out"=w120:dbl)
    n127 = feedback-in #16(w120) -> ()
    n128 = case shown="True" w85 {
      frame False {
        "Trip Relay6" <- TRUE ("Manual trip Relay1")
      }
      frame True {
        n129 = local write "Reclose Relay6?"(TRUE ("Reclose Relay1?")) -> ()
        n130 = local write "Trip Relay6"(FALSE ("Reclose Relay1?")) -> ()
      }
    }
    n131 = case shown="True" w89 {
      frame False {
        "Trip Relay2" <- TRUE ("Manual trip Relay1")
      }
      frame True {
        n132 = local write "Reclose Relay2?"(TRUE ("Reclose Relay1?")) -> ()
        n133 = local write "Trip Relay2"(FALSE ("Reclose Relay1?")) -> ()
      }
    }
    n134 = Index Array(array=w30) -> (element #2=w16:bool)  [unwired: 2 in, 1 out]
    n135 = Index Array(array=w29) -> (element #1=w25:bool, element #2=w15:bool)  [unwired: 2 in]
    n136 = Index Array(array=w28) -> (element #1=w23:bool, element #2=w14:bool)  [unwired: 2 in]
    n137 = Index Array(array=w27) -> (element #1=w20:bool, element #2=w13:bool)  [unwired: 2 in]
    n138 = Index Array(array=w26) -> (element #1=w18:bool)  [unwired: 2 in, 1 out]
    n139 = Build Array(w363, w364, w362, w361, w360, w359, w357, w356, w355, w355) -> (w106:dbl[])
    "R1 Data for\ncommunication" <- w106
    n140 = Build Array(w331, w330, w332, w333, w334, w335, w337, w338, w339, w339) -> (w105:dbl[])
    "R2 Data for\ncommunication" <- w105
    n141 = Build Array(w296, w297, w295, w294, w293, w292, w95, w290, w289, w289) -> (w104:dbl[])
    "R3 Data for\ncommunication" <- w104
    n142 = Build Array(w271, w270, w272, w273, w274, w275, w277, w278, w279, w279) -> (w103:dbl[])
    "R4 Data for\ncommunication" <- w103
    n143 = Build Array(w219, w220, w218, w217, w216, w215, w213, w212, w211, w211) -> (w102:dbl[])
    "R5 Data for\ncommunication" <- w102
    n144 = Build Array(w193, w192, w194, w195, w196, w197, w198, w199, w200, w200) -> (w101:dbl[])
    "R6 Data for\ncommunication" <- w101
    n145 = Build Array(w148, w149, w147, w57, w56, w58, w94, w146, w145, w145) -> (w100:dbl[])
    "R7 Data for\ncommunication" <- w100
    n146 = Build Array(w127, w126, w128, w129, w130, w131, w132, w133, w134, w134) -> (w99:dbl[])
    "R8 Data for\ncommunication" <- w99
    n147 = case shown="True" w152 {
      selector: w152 -> [_ w445]
      tunnel: w151 -> [w442 _]
      frame False {
        n148 = case shown="True" w442 {
          selector: w442 -> [_ w443]
          frame False {
          }
          frame True {
            n149 = local write "Relay7"(w443) -> ()
          }
        }
      }
      frame True {
        n150 = local read "Block Relay7"() -> (w444:bool)
        n151 = Not(x=w445) -> (.not. x?=w446:bool)
        n152 = local write "Reclose Relay7?"(w446) -> ()
        n153 = case shown="False" w444 {
          selector: w444 -> [w447 _]
          frame False {
            n154 = local write "Relay7"(w447) -> ()
          }
          frame True {
          }
        }
      }
    }
    n155 = case shown="True" w327 {
      selector: w327 -> [_ w473]
      tunnel: w328 -> [w471 _]
      frame False {
        n156 = case shown="True" w471 {
          selector: w471 -> [_ w472]
          frame False {
          }
          frame True {
            n157 = local write "Relay2"(w472) -> ()
          }
        }
      }
      frame True {
        n158 = local read "Block Relay2"() -> (w474:bool)
        n159 = Not(x=w473) -> (.not. x?=w475:bool)
        n160 = local write "Reclose Relay2?"(w475) -> ()
        n161 = case shown="False" w474 {
          selector: w474 -> [w476 _]
          frame False {
            n162 = local write "Relay2"(w476) -> ()
          }
          frame True {
          }
        }
      }
    }
    n163 = case shown="True" w123 {
      selector: w123 -> [_ w438]
      tunnel: w124 -> [w435 _]
      frame False {
        n164 = case shown="True" w435 {
          selector: w435 -> [_ w436]
          frame False {
          }
          frame True {
            n165 = local write "Relay8"(w436) -> ()
          }
        }
      }
      frame True {
        n166 = local read "Block Relay8"() -> (w437:bool)
        n167 = Not(x=w438) -> (.not. x?=w439:bool)
        n168 = case shown="False" w437 {
          selector: w437 -> [w440 _]
          frame False {
            n169 = local write "Relay8"(w440) -> ()
          }
          frame True {
          }
        }
        n170 = local write "Reclose Relay8?"(w439) -> ()
      }
    }
    n171 = case shown="True" w267 {
      selector: w267 -> [_ w464]
      tunnel: w268 -> [w460 _]
      frame False {
        n172 = case shown="True" w460 {
          selector: w460 -> [_ w461]
          frame False {
          }
          frame True {
            n173 = local write "Relay4"(w461) -> ()
          }
        }
      }
      frame True {
        n174 = local read "Block Relay4"() -> (w462:bool)
        n175 = Not(x=w464) -> (.not. x?=w463:bool)
        n176 = local write "Reclose Relay4?"(w463) -> ()
        n177 = case shown="False" w462 {
          selector: w462 -> [w465 _]
          frame False {
            n178 = local write "Relay4"(w465) -> ()
          }
          frame True {
          }
        }
      }
    }
    n179 = case shown="True" w223 {
      selector: w223 -> [_ w457]
      tunnel: w222 -> [w453 _]
      frame False {
        n180 = case shown="True" w453 {
          selector: w453 -> [_ w454]
          frame False {
          }
          frame True {
            n181 = local write "Relay5"(w454) -> ()
          }
        }
      }
      frame True {
        n182 = local read "Block Relay5"() -> (w455:bool)
        n183 = Not(x=w457) -> (.not. x?=w456:bool)
        n184 = local write "Reclose Relay5?"(w456) -> ()
        n185 = case shown="False" w455 {
          selector: w455 -> [w458 _]
          frame False {
            n186 = local write "Relay5"(w458) -> ()
          }
          frame True {
          }
        }
      }
    }
    n187 = case shown="True" w368 {
      tunnel: w367 -> [w552 _]
      frame False {
        n188 = case shown="True" w552 {
          selector: w552 -> [_ w553]
          frame False {
          }
          frame True {
            n189 = local write "Relay1"(w553) -> ()
          }
        }
      }
      frame True {
        w554 = FALSE ("Relay7")
        n190 = local write "Reclose Relay1?"(w554) -> ()
        n191 = local write "Relay1"(w554) -> ()
      }
    }
    n192 = case shown="True" w300 {
      tunnel: w299 -> [w467 _]
      frame False {
        n193 = case shown="True" w467 {
          selector: w467 -> [_ w468]
          frame False {
          }
          frame True {
            n194 = local write "Relay3"(w468) -> ()
          }
        }
      }
      frame True {
        w469 = FALSE ("Relay7")
        n195 = local write "Reclose Relay3?"(w469) -> ()
        n196 = local write "Relay3"(w469) -> ()
      }
    }
    n197 = case shown="True" w84 {
      frame False {
        "Trip Relay7" <- TRUE ("Manual trip Relay1")
      }
      frame True {
        n198 = local write "Reclose Relay7?"(TRUE ("Reclose Relay1?")) -> ()
        n199 = local write "Trip Relay7"(FALSE ("Reclose Relay1?")) -> ()
      }
    }
    n200 = case shown="False" w189 {
      tunnel: w190 -> [w449 _]
      frame False {
        n201 = case shown="True" w449 {
          selector: w449 -> [_ w450]
          frame False {
          }
          frame True {
            n202 = local write "Relay6"(w450) -> ()
          }
        }
      }
      frame True {
        w451 = FALSE ("Relay7")
        n203 = local write "Reclose Relay6?"(w451) -> ()
        n204 = local write "Relay6"(w451) -> ()
      }
    }
    n205 = case shown="False" w88 {
      frame False {
        "Trip Relay3" <- TRUE ("Reclose Relay1?")
      }
      frame True {
        n206 = local write "Reclose Relay3?"(TRUE ("Manual trip Relay1")) -> ()
        n207 = local write "Trip Relay3"(FALSE ("Manual trip Relay1")) -> ()
      }
    }
    n208 = feedback #17() -> (w393:bool)  [unwired: 1 in]
    n209 = feedback-in #17("Manual trip Relay1") -> ()
    n210 = feedback #18() -> (w255:bool)  [unwired: 1 in]
    n211 = feedback-in #18("Manual trip Relay4") -> ()
    n212 = feedback #19() -> (w235:bool)  [unwired: 1 in]
    n213 = feedback-in #19("Manual trip Relay5") -> ()
    n214 = feedback #20() -> (w177:bool)  [unwired: 1 in]
    n215 = feedback-in #20("Manual trip Relay6") -> ()
    n216 = feedback #21() -> (w111:bool)  [unwired: 1 in]
    n217 = feedback-in #21("Manual trip Relay8") -> ()
    n218 = feedback #22() -> (w164:bool)  [unwired: 1 in]
    n219 = feedback-in #22("Manual trip Relay7") -> ()
    n220 = feedback #23() -> (w315:bool)  [unwired: 1 in]
    n221 = feedback-in #23("Manual trip Relay2") -> ()
    n222 = Compound Arithmetic op=OR(w25, w23, w20, w18) -> (→"Block Relay2":bool)
    n223 = Compound Arithmetic op=OR(w16, w23, w20, w18) -> (→"Block Relay4":bool)
    n224 = Compound Arithmetic op=OR(w16, w15, w14, w18) -> (→"Block Relay7":bool)
    n225 = Compound Arithmetic op=OR(w16, w15, w20, w18) -> (→"Block Relay5":bool)
    n226 = Compound Arithmetic op=OR(w16, w15, w14, w13) -> (→"Block Relay8":bool)
    n227 = feedback #24() -> (w312:bool)  [unwired: 1 in]
    n228 = feedback-in #24("Manual trip Relay3") -> ()
    n229 = local read "Trip Relay8"() -> (w81:bool)
    n230 = local read "Trip Relay2"() -> (w69:bool)
    n231 = local read "Trip Relay7"() -> (w79:bool)
    n232 = local read "Trip Relay5"() -> (w75:bool)
    n233 = local read "Trip Relay1"() -> (w67:bool)
    n234 = local read "Trip Relay3"() -> (w71:bool)
    n235 = local read "Trip Relay4"() -> (w73:bool)
    n236 = local read "Trip Relay6"() -> (w77:bool)
    n237 = Not Equal?(x="Manual trip Relay1", y=w393) -> (x != y?=w392:bool)
    n238 = Not Equal?(x="Manual trip Relay4", y=w255) -> (x != y?=w256:bool)
    n239 = Not Equal?(x="Manual trip Relay5", y=w235) -> (x != y?=w234:bool)
    n240 = Not Equal?(x="Manual trip Relay6", y=w177) -> (x != y?=w178:bool)
    n241 = Not Equal?(x="Manual trip Relay8", y=w111) -> (x != y?=w112:bool)
    n242 = Not Equal?(x="Manual trip Relay7", y=w164) -> (x != y?=w163:bool)
    n243 = Not Equal?(x="Manual trip Relay2", y=w315) -> (x != y?=w316:bool)
    n244 = Not Equal?(x="Manual trip Relay3", y=w312) -> (x != y?=w311:bool)
    n245 = And(x="Manual trip Relay1", y=w392) -> (x .and. y?=w390:bool)
    n246 = And(x="Manual trip Relay4", y=w256) -> (x .and. y?=w258:bool)
    n247 = And(x="Manual trip Relay5", y=w234) -> (x .and. y?=w232:bool)
    n248 = And(x="Manual trip Relay6", y=w178) -> (x .and. y?=w180:bool)
    n249 = And(x="Manual trip Relay8", y=w112) -> (x .and. y?=w114:bool)
    n250 = And(x="Manual trip Relay7", y=w163) -> (x .and. y?=w161:bool)
    n251 = And(x="Manual trip Relay2", y=w316) -> (x .and. y?=w318:bool)
    n252 = And(x="Manual trip Relay3", y=w311) -> (x .and. y?=w309:bool)
    n253 = Or(x=w232, y=w75) -> (x .or. y?=w76:bool)
    n254 = Or(x=w390, y=w67) -> (x .or. y?=w68:bool)
    n255 = Or(x=w161, y=w79) -> (x .or. y?=w80:bool)
    n256 = Or(x=w258, y=w73) -> (x .or. y?=w74:bool)
    n257 = Or(x=w180, y=w77) -> (x .or. y?=w78:bool)
    n258 = Or(x=w318, y=w69) -> (x .or. y?=w70:bool)
    n259 = Or(x=w309, y=w71) -> (x .or. y?=w72:bool)
    n260 = Or(x=w114, y=w81) -> (x .or. y?=w82:bool)
    n261 = case shown="True" w83 {
      frame False {
        "Trip Relay8" <- TRUE ("Manual trip Relay1")
      }
      frame True {
        n262 = local write "Reclose Relay8?"(TRUE ("Reclose Relay1?")) -> ()
        n263 = local write "Trip Relay8"(FALSE ("Reclose Relay1?")) -> ()
      }
    }
    n264 = case shown="True" w76 {
      frame False {
      }
      frame True {
        w459 = FALSE ("Relay7")
        n265 = local write "Reclose Relay5?"(w459) -> ()
        n266 = local write "Relay5"(w459) -> ()
      }
    }
    n267 = case shown="True" w87 {
      frame False {
        "Trip Relay4" <- TRUE ("Manual trip Relay1")
      }
      frame True {
        n268 = local write "Reclose Relay4?"(TRUE ("Reclose Relay1?")) -> ()
        n269 = local write "Trip Relay4"(FALSE ("Trip Relay4")) -> ()
      }
    }
    n270 = case shown="True" w68 {
      frame False {
      }
      frame True {
        w555 = FALSE ("Relay7")
        n271 = local write "Reclose Relay1?"(w555) -> ()
        n272 = local write "Relay1"(w555) -> ()
      }
    }
    n273 = case shown="True" w74 {
      frame False {
      }
      frame True {
        w466 = FALSE ("Relay7")
        n274 = local write "Reclose Relay4?"(w466) -> ()
        n275 = local write "Relay4"(w466) -> ()
      }
    }
    n276 = case shown="True" w78 {
      frame False {
      }
      frame True {
        w452 = FALSE ("Relay7")
        n277 = local write "Reclose Relay6?"(w452) -> ()
        n278 = local write "Relay6"(w452) -> ()
      }
    }
    n279 = case shown="True" w80 {
      frame False {
      }
      frame True {
        w448 = FALSE ("Relay7")
        n280 = local write "Reclose Relay7?"(w448) -> ()
        n281 = local write "Relay7"(w448) -> ()
      }
    }
    n282 = case shown="True" w72 {
      frame False {
      }
      frame True {
        w470 = FALSE ("Relay7")
        n283 = local write "Reclose Relay3?"(w470) -> ()
        n284 = local write "Relay3"(w470) -> ()
      }
    }
    n285 = case shown="True" w82 {
      frame False {
      }
      frame True {
        w441 = FALSE ("Relay7")
        n286 = local write "Reclose Relay8?"(w441) -> ()
        n287 = local write "Relay8"(w441) -> ()
      }
    }
    n288 = case shown="True" w70 {
      frame False {
      }
      frame True {
        w477 = FALSE ("Relay7")
        n289 = local write "Reclose Relay2?"(w477) -> ()
        n290 = local write "Relay2"(w477) -> ()
      }
    }
    n291 = Subtract(x=w57, y=w56) -> (x-y=w55:dbl)
    n292 = Build Array (concatenate)(w106, w105, w104, w103, w102, w101, w100, w99) -> (w107:dbl[])
    n293 = shared-variable "IntelliRupter\\IntelliRupter_data.lvlib\\Relay7_Ang_Diff"(w58) -> ()  [unwired: 1 in, 1 out]
    n294 = shared-variable "IntelliRupter\\IntelliRupter_data.lvlib\\Relay7_Freq_Diff"(w55) -> ()  [unwired: 1 in, 1 out]
    n295 = shared-variable "IntelliRupter\\IntelliRupter_data.lvlib\\Relay_to_MGCC"(w107) -> ()  [unwired: 1 in, 1 out]
    n296 = shared-variable "IntelliRupter\\IntelliRupter_data.lvlib\\Relay7_Cmd"("Relay7") -> ()  [unwired: 1 in, 1 out]
    n297 = xnode "Read/Write Control"("FPGA VI Reference In"=w389, "Relay1"="Relay1", "Relay2"="Relay2", "Relay3"="Relay3", "Relay4"="Relay4", "Relay5"="Relay5", "Relay6"="Relay6", "Relay7"="Relay7", "Relay8"="Relay8", "Count(ticks)"="Count(ticks)") -> ("FPGA VI Reference Out"=w395:refnum<k20>, "error out"=w394:errorcluster)  [unwired: 1 in]
  }
  n298 = xnode "Close FPGA VI Reference"("FPGA VI Reference In"=w9, "error in"=w8) -> ()  [unwired: 1 out]
